vi "qLST.vi"(0 "System no.":i32=1 min=1 max=4 step=1, 5 "error in":errorcluster) -> (14 "File Name":string[](array[string]), 15 "File Size":u32[](array[numeric]), 19 "error out":errorcluster)   [LabVIEW 2026]
doc: "Lists names of data files in nonvolatile memory.\n\nE-754: Check HLP? answer to find out if LST? is supported"
panel:
  # "Lists names of data files in nonvolatile memory."
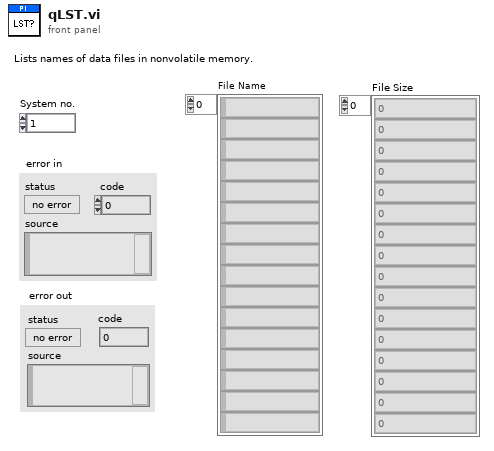
[diagram p1: front panel]
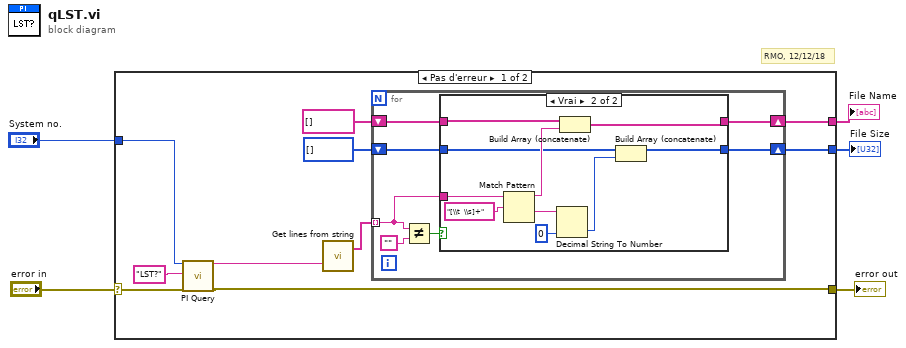
[diagram p0: block diagram]
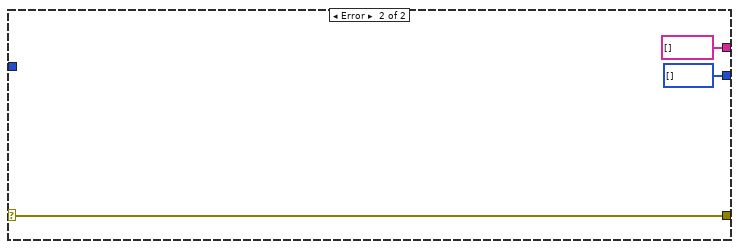
[diagram p3: hidden frame]
diagram:
  # "RMO, 12/12/18"
  n1 = case shown="Pas d'erreur" "error in" {
    selector: "error in" -> [w15 w37]
    tunnel: [w6 w37] -> w5
    tunnel: "System no." -> [w13 _]
    tunnel: [w9 string[] []] -> w2
    tunnel: [w8 u32[] []] -> w1
    frame No Error {
      n2 = call "PI Query.vi"("System no."=w13, "String to send"="LST?", "error in"=w15) -> ("String read"=w7:string, "error out"=w6:errorcluster)  [unwired: 4 in, 11 out]
      n3 = call "Get lines from string.vi"("Input string"=w7) -> ("Strings"=w12:string[])  [unwired: 2 in, 16 out]
      n4 = for {
        tunnel: w12 -> [w20] mode=indexing
        shift-right: [w17] -> w9
        shift-left: string[] [] -> [w19]
        shift-right: [w16] -> w8
        shift-left: u32[] [] -> [w18]
        n5 = Not Equal?(x=w20, y="") -> (x != y?=w21:bool)
        n6 = case shown="Vrai" w21 {
          tunnel: w20 -> [_ w34]
          tunnel: w19 -> [w24 w32]
          tunnel: w18 -> [w23 w29]
          tunnel: [w24 w30] -> w17
          tunnel: [w23 w28] -> w16
          frame False {
            # "empty string"
          }
          frame True {
            n7 = Match Pattern(string=w34, regular expression="[\\t  \\s]+") -> (before substring=w31:string, after substring=w27:string)  [unwired: 3 out]
            n8 = Decimal String To Number(string=w27, default (0L)=u32 0) -> (number=w25:u32)  [unwired: 2 out]
            n9 = Build Array (concatenate)(w32, w31) -> (w30:string[])
            n10 = Build Array (concatenate)(w29, w25) -> (w28:u32[])
          }
        }
      }
    }
    frame Error {
    }
  }
  "error out" <- w5
  "File Name" <- w2
  "File Size" <- w1
